vi "svx_Property Page.vi"(6 "Z Scale Graph Refnum":refnum<vi>, 7 "XY Graph Reference":refnum<vi>, 8 "XY Scale Graph Refnum":refnum<vi>, 9 "Container Refnum":refnum<vi>, 10 "State in":T1={"X Scale Width %"=50.0, "Y Scale Height %"=50.0, "X-Axis Range"={"Minimum"=0.0, "Maximum"=10.0}, "Y-Axis Range"={"Minimum"=0.0, "Maximum"=10.0}, "Z-Axis Range"={"Minimum"=0.0, "Maximum"=10.0}, "Plot Color"=61212, "Frame Color"=16252785, "Background Color"=16777222, "Initial AutoScale Y"=TRUE, "AutoScale X"=2, "AutoScale Y"=2, "AutoScale Z"=2, "Plot Transparency"=FALSE, "X-Axis Name"="Frequency", "Y-Axis Name"="Amplitude", "Z-Axis Name"="", "X-Axis Scaling Factor"={"Offset"=0.0, "Multiplier"=1.0}, "Y-Axis Scaling Factor"={"Offset"=0.0, "Multiplier"=1.0}, "Z-Axis Scaling Factor"={"Offset"=0.0, "Multiplier"=1.0}, "X-Scale Visible"=TRUE, "Y-Scale Visible"=TRUE, "Z-Scale Visible"=TRUE, "X-Scale Label Visible"=TRUE, "Y-Scale Label Visible"=TRUE, "Z-Scale Label Visible"=TRUE, "X-Axis Range Scaled"={"Minimum"=0.0, "Maximum"=10.0}, "Y-Axis Range Scaled"={"Minimum"=0.0, "Maximum"=10.0}, "Z-Axis Range Scaled"={"Minimum"=0.0, "Maximum"=10.0}, "Rev Z Order"=FALSE, "X-Scale Format Str"="%#.4g", "Y-Scale Format Str"="%#.4g", "Z-Scale Format Str"="%#.4g", "Decor color"=12369084, "Scale Range Change"=refnum, "out of state queue"=refnum, "property nodes"=refnum, "Lines"=[], "Line Properties"={"Line Color"=61212, "Line Width"=61212, "Line Style"=enum."Dash", "DisplayLines"=FALSE}} caption="State" {"Line Properties"."Line Width" min=1}, 11 "Data In":T3={"z0"=0.0, "dz"=1.0, "Plots"=[]}) -> (1 "Cancel?":bool, 2 "State out":T1={"X Scale Width %"=50.0, "Y Scale Height %"=50.0, "X-Axis Range"={"Minimum"=0.0, "Maximum"=10.0}, "Y-Axis Range"={"Minimum"=0.0, "Maximum"=10.0}, "Z-Axis Range"={"Minimum"=0.0, "Maximum"=10.0}, "Plot Color"=61212, "Frame Color"=16252785, "Background Color"=16777222, "Initial AutoScale Y"=TRUE, "AutoScale X"=2, "AutoScale Y"=2, "AutoScale Z"=2, "Plot Transparency"=FALSE, "X-Axis Name"="Frequency", "Y-Axis Name"="Amplitude", "Z-Axis Name"="", "X-Axis Scaling Factor"={"Offset"=0.0, "Multiplier"=1.0}, "Y-Axis Scaling Factor"={"Offset"=0.0, "Multiplier"=1.0}, "Z-Axis Scaling Factor"={"Offset"=0.0, "Multiplier"=1.0}, "X-Scale Visible"=TRUE, "Y-Scale Visible"=TRUE, "Z-Scale Visible"=TRUE, "X-Scale Label Visible"=TRUE, "Y-Scale Label Visible"=TRUE, "Z-Scale Label Visible"=TRUE, "X-Axis Range Scaled"={"Minimum"=0.0, "Maximum"=10.0}, "Y-Axis Range Scaled"={"Minimum"=0.0, "Maximum"=10.0}, "Z-Axis Range Scaled"={"Minimum"=0.0, "Maximum"=10.0}, "Rev Z Order"=FALSE, "X-Scale Format Str"="%#.4g", "Y-Scale Format Str"="%#.4g", "Z-Scale Format Str"="%#.4g", "Decor color"=12369084, "Scale Range Change"=refnum, "out of state queue"=refnum, "property nodes"=refnum, "Lines"=[], "Line Properties"={"Line Color"=61212, "Line Width"=61212, "Line Style"=enum."Dash", "DisplayLines"=FALSE}} caption="State" {"Line Properties"."Line Width" min=1})   [LabVIEW 2017, in "SVX Waterfall Graph.xctl"]
uses:
  <vilib>/addons/_XControls/Waterfall Graph/SVX Waterfall Graph.xctl
  <vilib>/addons/_XControls/Waterfall Graph/subVIs/svx_Waterfall Data.ctl
  <vilib>/addons/_XControls/Waterfall Graph/subVIs/svx_Waterfall State.ctl
  <vilib>/addons/_NISVFA/_Shared subVIs/Controls/svc_Cluster of Array of Cluster of XYZ.ctl
  <vilib>/addons/_XControls/Waterfall Graph/subVIs/svx_Waterfall Property Page User Events.ctl
panel:
  in  "Help":bool
  in  "Cancel":bool
  in  "OK":bool
  in  "Tab Control":T4(tab)
  in  "Reverse Order":bool
  in  "Plot Transparency":bool
  in  "Background color":u32(colorbox)
  in  "Frame color":u32(colorbox)
  in  "Plot color":u32(colorbox)
  in  "Enable State":T5(radio)
  in  "Caption":string
  in  "Label":string
  in  "Caption Visible?":bool
  in  "Label Visible?":bool
  in  "trailing zeros":bool
  in  "Digits":u8=1
  in  "Precision Type":u16(ring) caption="Precision type" items=["Digits of precision", "Significant digits"]
  in  "Type":i32(listbox)
  in  "FP Axis":enum16{"X-Axis", "Y-Axis", "Z-Axis"}(ring)
  in  "Scaling Factors - Multiplier":dbl caption="Multiplier"
  in  "Scaling Factors - Offset":dbl caption="Offset"
  in  "Range Maximum":dbl caption="Maximum"
  in  "Range Minimum":dbl caption="Minimum"
  in  "Autoscale":bool
  in  "Show Scale":bool
  in  "Show Scale label":bool
  in  "Scale Name":string caption="Name"
  in  "Scale Axis":enum16{"X-Axis", "Y-Axis", "Z-Axis"}(ring)
  in  "Line color":u32(colorbox)
  in  "Line width":u16=1 min=1 max=5
  in  "Style":T6(ring)=enum."Dash"
  in  "DisplayLines":bool
  in  "Tip strip":string
  in  "Description":string
  # "Label"
  # "Caption"
  # "Enabled State"
  # "Color Scheme"
  # "Scaling factors"
  # "Line Settings"
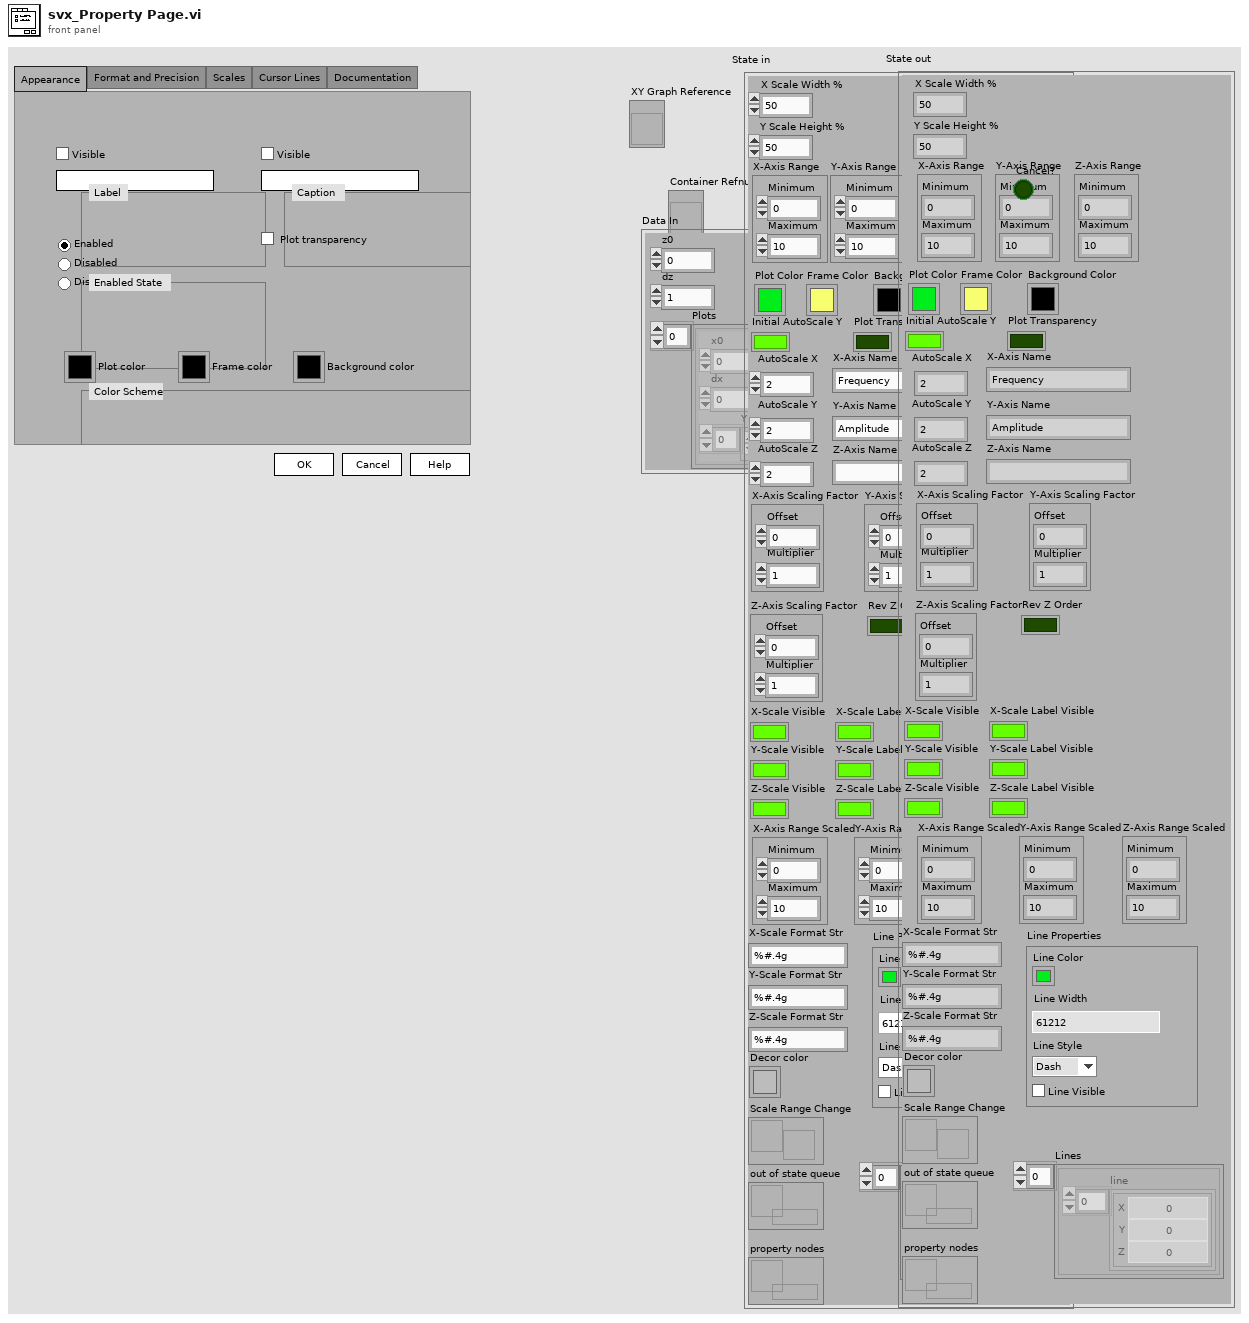
[diagram p1: front panel]
types:
  T1 = typedef "SVX Waterfall Graph.xctl/svx_Waterfall State.ctl" = cluster{"X Scale Width %":dbl, "Y Scale Height %":dbl, "X-Axis Range":cluster{"Minimum":dbl, "Maximum":dbl}, "Y-Axis Range":cluster{"Minimum":dbl, "Maximum":dbl}, "Z-Axis Range":cluster{"Minimum":dbl, "Maximum":dbl}, "Plot Color":u32, "Frame Color":u32, "Background Color":u32, "Initial AutoScale Y":bool, "AutoScale X":u8, "AutoScale Y":u8, "AutoScale Z":u8, "Plot Transparency":bool, "X-Axis Name":string, "Y-Axis Name":string, "Z-Axis Name":string, "X-Axis Scaling Factor":cluster{"Offset":dbl, "Multiplier":dbl}, "Y-Axis Scaling Factor":cluster{"Offset":dbl, "Multiplier":dbl}, "Z-Axis Scaling Factor":cluster{"Offset":dbl, "Multiplier":dbl}, "X-Scale Visible":bool, "Y-Scale Visible":bool, "Z-Scale Visible":bool, "X-Scale Label Visible":bool, "Y-Scale Label Visible":bool, "Z-Scale Label Visible":bool, "X-Axis Range Scaled":cluster{"Minimum":dbl, "Maximum":dbl}, "Y-Axis Range Scaled":cluster{"Minimum":dbl, "Maximum":dbl}, "Z-Axis Range Scaled":cluster{"Minimum":dbl, "Maximum":dbl}, "Rev Z Order":bool, "X-Scale Format Str":string, "Y-Scale Format Str":string, "Z-Scale Format Str":string, "Decor color":u32, "Scale Range Change":refnum<user-event>, "out of state queue":refnum<queue>, "property nodes":refnum<queue>, "Lines":T2[], "Line Properties":cluster{"Line Color":u32, "Line Width":u16, "Line Style":enum32{"Solid", "Dash", "Dot", "DashDot", "DashDotDot"}, "DisplayLines":bool}}
  T2 = typedef "svc_Cluster of Array of Cluster of XYZ.ctl" = cluster{"line":cluster{"X":dbl, "Y":dbl, "Z":dbl}[]}
  T3 = typedef "SVX Waterfall Graph.xctl/svx_Waterfall Data.ctl" = cluster{"z0":dbl, "dz":dbl, "Plots":cluster{"x0":dbl, "dx":dbl, "Y":dbl[]}[]}
  T4 = enum32{"Appearance", "Format and Precision", "Scales", "Cursor Lines", "Documentation"}
  T5 = enum32{"Enabled", "Disabled", "Disabled & grayed"}
  T6 = enum32{"Solid", "Dash", "Dot", "DashDot", "DashDotDot"}
  T7 = typedef "SVX Waterfall Graph.xctl/svx_Waterfall Property Page User Events.ctl" = enum16{"Redraw Frame", "Update Graph", "Exit"}
  T8 = cluster{"Container Changed":bool, "Scales Changed":bool, "Waveform Changed":bool}
  T9 = cluster{"Line Color":u32, "Line Width":u16, "Line Style":enum32{"Solid", "Dash", "Dot", "DashDot", "DashDotDot"}, "DisplayLines":bool}
  T10 = cluster{"Label.Text":string, "Label.Visible":bool, "Caption.Text":string, "Caption.Visible":bool, "Disabled":u8, "Desc":string, "TipStrip":string}
  T11 = cluster{"Width":u16, "Style":enum32{"Solid", "Dash", "Dot", "DashDot", "DashDotDot"}}
  T12 = typedef "SVX Waterfall Graph.xctl/svx_CroppedData.ctl" = cluster{"Dec/Cropped in":T3, "Lines":T2[]}
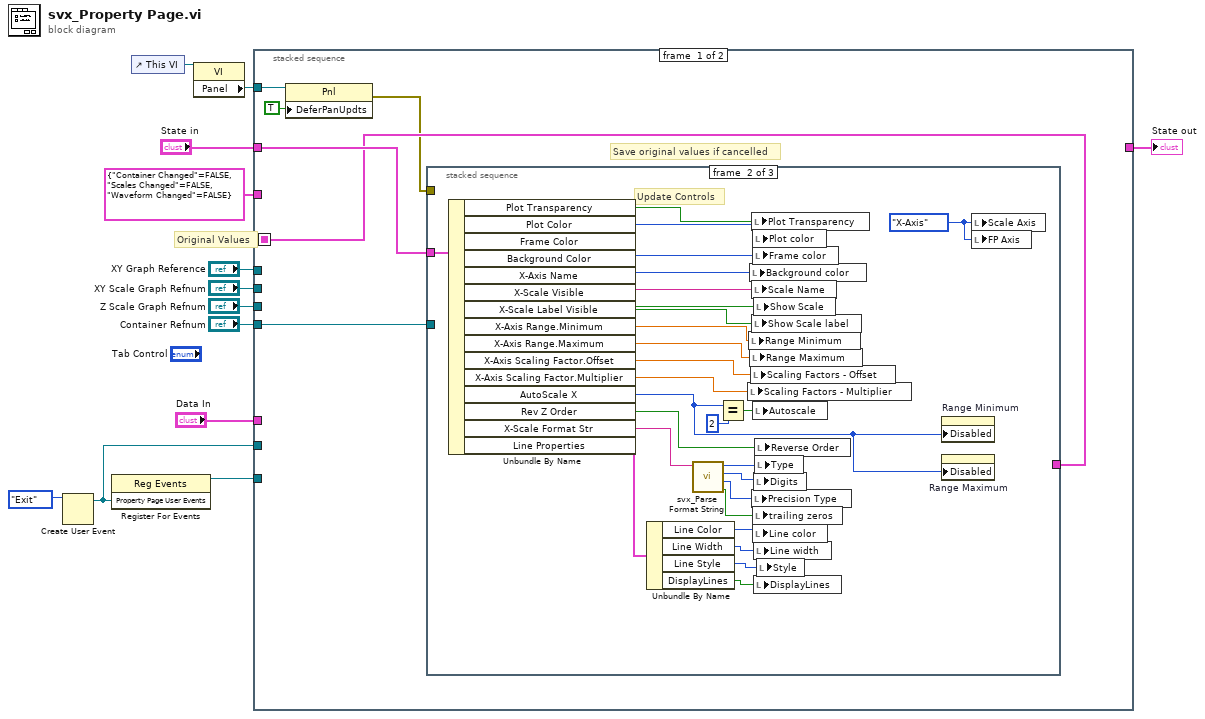
[diagram p0: block diagram]
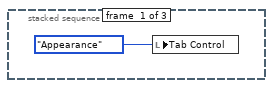
[diagram p2: hidden frame]
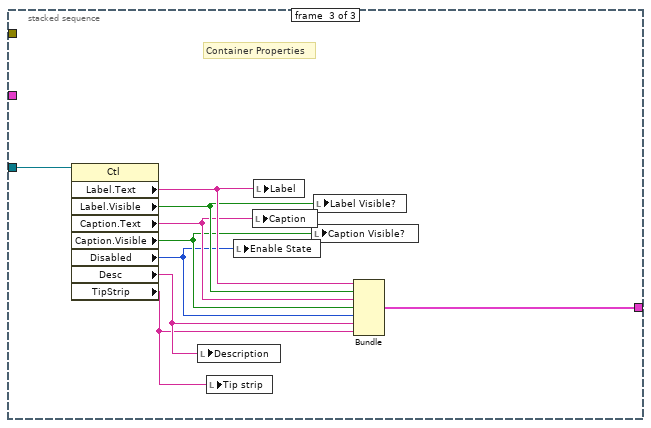
[diagram p3: hidden frame]
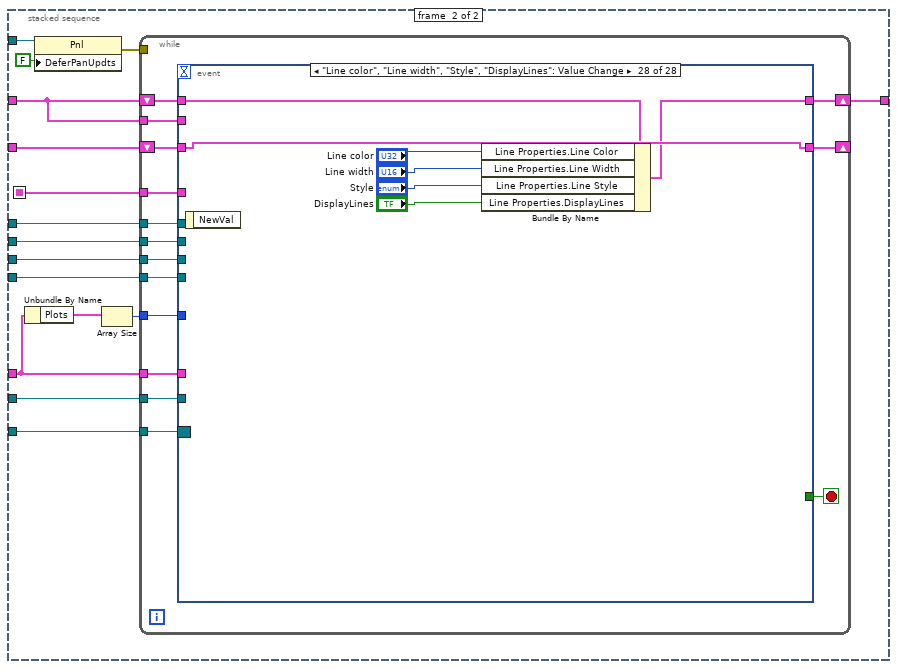
[diagram p4: hidden frame]
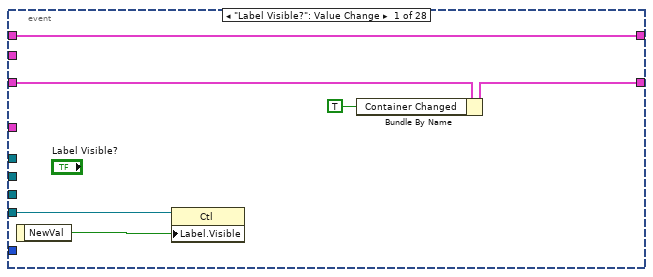
[diagram p5: hidden frame]
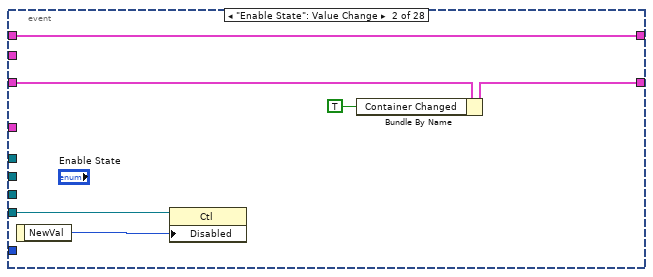
[diagram p6: hidden frame]
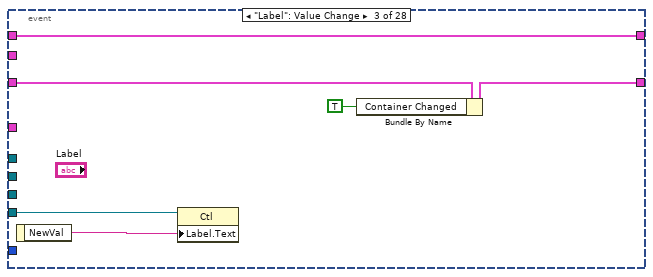
[diagram p7: hidden frame]
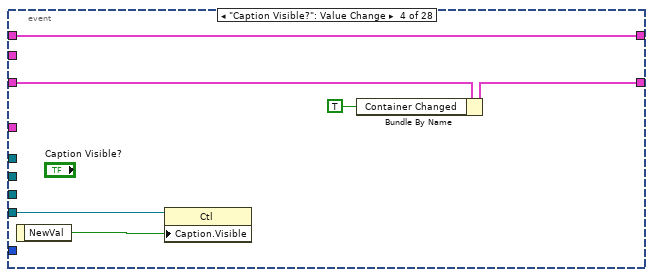
[diagram p8: hidden frame]
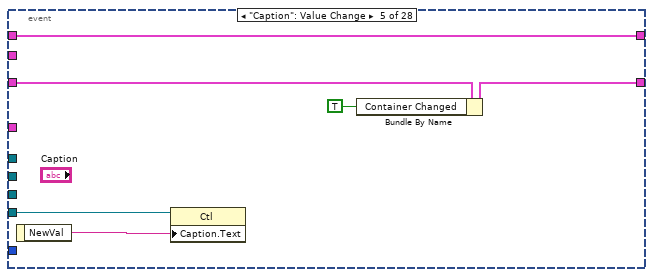
[diagram p9: hidden frame]
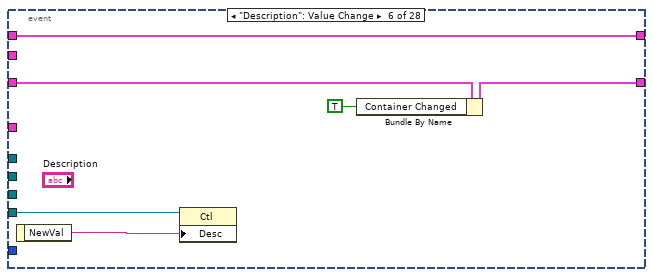
[diagram p10: hidden frame]
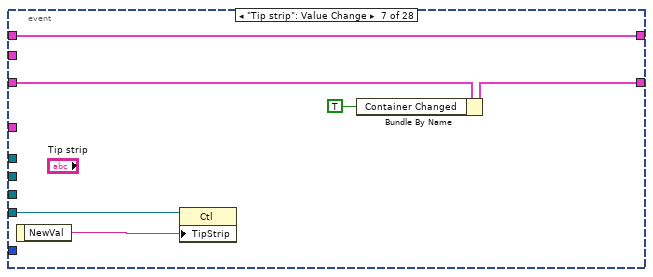
[diagram p11: hidden frame]
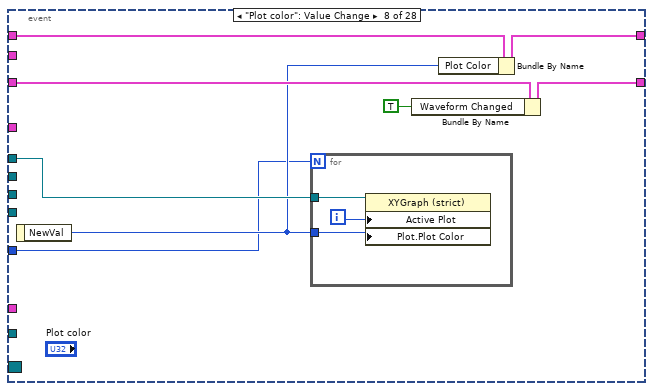
[diagram p12: hidden frame]
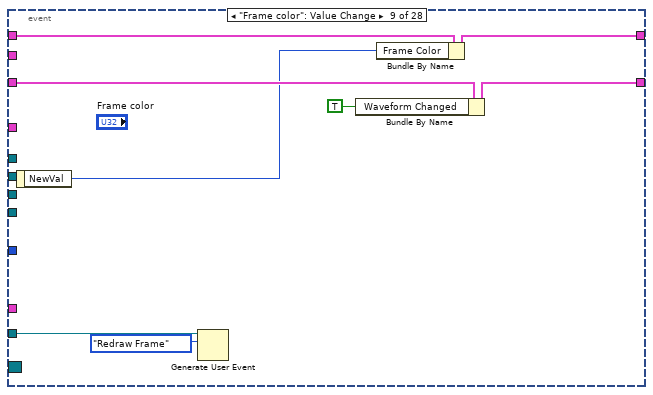
[diagram p13: hidden frame]
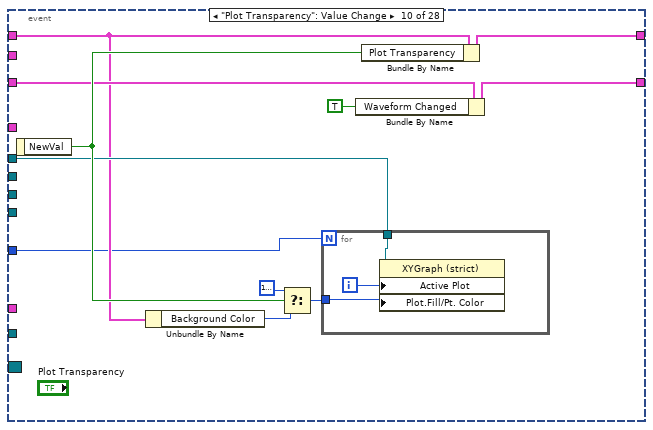
[diagram p14: hidden frame]
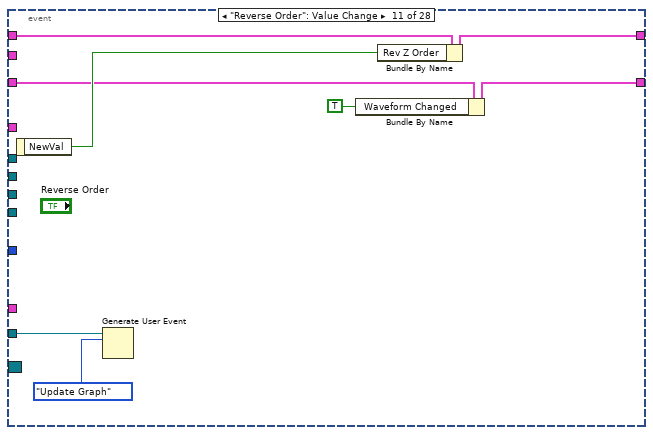
[diagram p15: hidden frame]
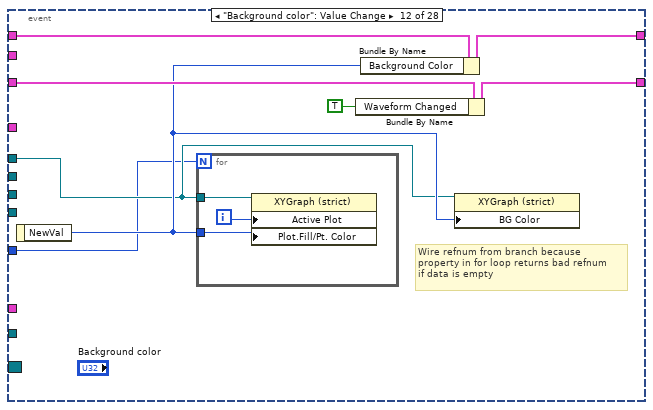
[diagram p16: hidden frame]
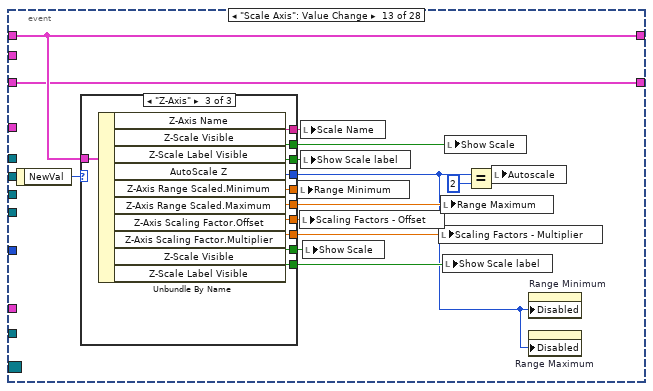
[diagram p17: hidden frame]
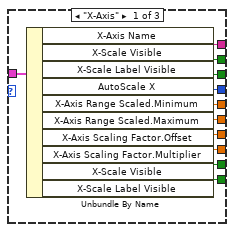
[diagram p18: hidden frame]
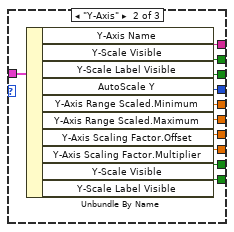
[diagram p19: hidden frame]
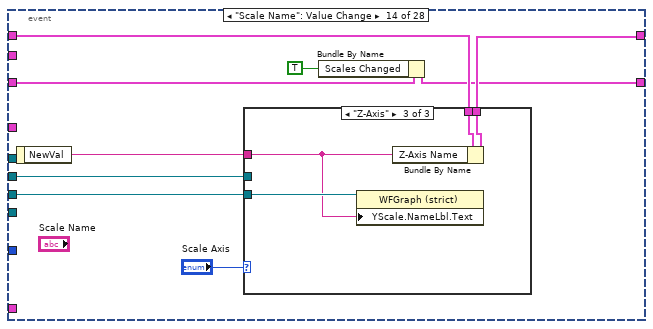
[diagram p20: hidden frame]
diagram:
  # "Original Values"
  n1 = Create User Event(user event datatype=svx_Waterfall_Property_Page_User_Events."Exit" ("Property Page User Events")) -> (user event=w4:refnum<user-event>)  [unwired: 1 in, 1 out]
  n2 = register-events(w4) -> (reference out=w6:refnum<event-registration>)  [unwired: 2 in, 1 out]
  n3 = control-ref of="This VI"() -> (w2:refnum<vi>)
  n4 = property class="VI"(reference=w2) -> ("Panel"=w1:refnum<vi>)  [unwired: 1 in, 2 out]
  n5 = stacked-sequence {
    seq-local: [w17 _] -> [_ w65]
    tunnel: T8 {"Container Changed"=FALSE, "Scales Changed"=FALSE, "Waveform Changed"=FALSE} -> [_ w72]
    tunnel: "XY Graph Reference" -> [_ w71]
    tunnel: "XY Scale Graph Refnum" -> [_ w70]
    tunnel: "Z Scale Graph Refnum" -> [_ w69]
    tunnel: "Container Refnum" -> [w19 w68]
    tunnel: "State in" -> [w18 w66]
    tunnel: [_ w67] -> w8
    tunnel: "Data In" -> [_ w58]
    tunnel: w6 -> [_ w64]
    tunnel: w4 -> [_ w63]
    tunnel: w1 -> [w16 w61]
    frame #0 {
      # "Save original values if cancelled"
      n6 = property class="Pnl"(reference=w16, "DeferPanUpdts"=TRUE ("Defer Panel Updates")) -> (error out=w14:errorcluster)  [unwired: 1 in, 1 out]
      n7 = stacked-sequence {
        tunnel: w19 -> [_ _ w56]
        tunnel: [_ _ w55] -> w17
        tunnel: w18 -> [_ w47 _]
        tunnel: w14 -> [_ _ _]
        frame #0 {
          n8 = local write "Tab Control"(T4."Appearance" ("Tab Control")) -> ()
        }
        frame #1 {
          w32 = enum16{"X-Axis", "Y-Axis", "Z-Axis"}."X-Axis" ("Axis")
          # "Update Controls"
          n9 = Unbundle By Name(w47) -> ("Plot Transparency"=w37:bool, "Plot Color"=w46:u32, "Frame Color"=w45:u32, "Background Color"=w44:u32, "X-Axis Name"=w43:string, "X-Scale Visible"=w42:bool, "X-Scale Label Visible"=w41:bool, "X-Axis Range.Minimum"=w40:dbl, "X-Axis Range.Maximum"=w26:dbl, "X-Axis Scaling Factor.Offset"=w39:dbl, "X-Axis Scaling Factor.Multiplier"=w38:dbl, "AutoScale X"=w36:u8, "Rev Z Order"=w33:bool, "X-Scale Format Str"=w31:string, "Line Properties"=w25:T9)
          n10 = Unbundle By Name(w25) -> ("Line Color"=w24:u32, "Line Width"=w23:u16, "Line Style"=w22:T6, "DisplayLines"=w21:bool)
          n11 = call <vilib>:"svx_Parse Format String.vi"("Format string"=w31) -> ("trailing zeros"=w27:bool, "Precision Type"=w28:u16, "Digits"=w29:u8, "Type"=w30:i32)  [unwired: 6 in, 1 out]
          n12 = Equal?(x=w36, y=u8 2) -> (x = y?=w34:bool)
          n13 = local write "Scaling Factors - Multiplier"(w38) -> ()
          n14 = local write "Range Minimum"(w40) -> ()
          n15 = local write "Background color"(w44) -> ()
          n16 = local write "Range Maximum"(w26) -> ()
          n17 = local write "Scaling Factors - Offset"(w39) -> ()
          n18 = local write "Plot Transparency"(w37) -> ()
          n19 = local write "Scale Name"(w43) -> ()
          n20 = local write "Show Scale label"(w41) -> ()
          n21 = local write "Precision Type"(w28) -> ()
          n22 = local write "Plot color"(w46) -> ()
          n23 = local write "Frame color"(w45) -> ()
          n24 = local write "Autoscale"(w34) -> ()
          n25 = local write "trailing zeros"(w27) -> ()
          n26 = local write "Line color"(w24) -> ()
          n27 = local write "Show Scale"(w42) -> ()
          n28 = local write "Digits"(w29) -> ()
          n29 = local write "Line width"(w23) -> ()
          n30 = local write "DisplayLines"(w21) -> ()
          n31 = local write "Reverse Order"(w33) -> ()
          n32 = local write "Type"(w30) -> ()
          n33 = local write "Style"(w22) -> ()
          n34 = property on="Range Minimum" class="DigNum (strict)"("Disabled"=w36) -> ()  [unwired: 2 in, 2 out]
          n35 = property on="Range Maximum" class="DigNum (strict)"("Disabled"=w36) -> ()  [unwired: 2 in, 2 out]
          n36 = local write "Scale Axis"(w32) -> ()
          n37 = local write "FP Axis"(w32) -> ()
        }
        frame #2 {
          # "Container Properties"
          n38 = property class="Ctl"(reference=w56) -> ("Label.Text"=w54:string, "Label.Visible"=w53:bool, "Caption.Text"=w52:string, "Caption.Visible"=w51:bool, "Disabled"=w50:u8, "Desc"=w49:string, "TipStrip"=w48:string)  [unwired: 1 in, 2 out]
          n39 = local write "Description"(w49) -> ()
          n40 = local write "Tip strip"(w48) -> ()
          n41 = local write "Enable State"(w50) -> ()
          n42 = local write "Caption"(w52) -> ()
          n43 = local write "Label"(w54) -> ()
          n44 = local write "Caption Visible?"(w51) -> ()
          n45 = local write "Label Visible?"(w53) -> ()
          n46 = Bundle("Label.Text"=w54, "Label.Visible"=w53, "Caption.Text"=w52, "Caption.Visible"=w51, "Disabled"=w50, "Desc"=w49, "TipStrip"=w48) -> (w55:T10)  [unwired: 1 in]
        }
      }
    }
    frame #1 {
      n47 = Unbundle By Name(w58) -> ("Plots"=w59:cluster{"x0":dbl, "dx":dbl, "Y":dbl[]}[])
      n48 = property class="Pnl"(reference=w61, "DeferPanUpdts"=FALSE ("Defer Panel Updates")) -> (error out=w60:errorcluster)  [unwired: 1 in, 1 out]
      n49 = Array Size(array=w59) -> (size(s)=w57:i32)
      n50 = while {
        shift-right: [w85] -> _
        shift-left: w72 -> [w86]
        tunnel: w71 -> [w84]
        tunnel: w70 -> [w83]
        tunnel: w69 -> [w82]
        tunnel: w68 -> [w81]
        shift-right: [w79] -> w67
        shift-left: w66 -> [w80]
        tunnel: w66 -> [w78]
        tunnel: w65 -> [w77]
        tunnel: w58 -> [w76]
        tunnel: w64 -> [w75]
        tunnel: w63 -> [w74]
        tunnel: w60 -> [_]
        tunnel: w57 -> [w73]
        stop <- w87 stop-if-true
        n51 = event shown="[27] \"Line color\", \"Line width\", \"Style\", \"DisplayLines\": Value Change" {
          selector: w75 -> [_ _ _ _ _ _ _ _ _ _ _ _ _ _ _ _ _ _ _ _ _ _ _ _ _ _ _ _]
          dyn-events: _ -> [_ _ _ _ _ _ _ _ _ _ _ _ _ _ _ _ _ _ _ _ _ _ _ _ _ _ _ _]
          timeout: _ -> [_ _ _ _ _ _ _ _ _ _ _ _ _ _ _ _ _ _ _ _ _ _ _ _ _ _ _ _]
          tunnel: [_ _ _ _ _ _ _ _ _ _ _ _ _ _ _ _ _ _ _ _ _ _ _ w556 _ _ w652 _] -> w87
          tunnel: w86 -> [w93 w99 w105 w111 w117 w123 w129 w137 w148 w153 w166 w178 w187 w231 w253 w274 w295 w346 w403 w451 w502 w521 w542 w560 w569 w644 w654 w734]
          tunnel: [w92 w98 w104 w110 w116 w122 w128 w136 w147 w159 w170 w177 w187 w230 w252 w273 w294 w345 w402 w450 w501 w521 w541 w560 w569 w644 w654 w734] -> w85
          tunnel: w84 -> [_ _ _ _ _ _ _ w134 _ w151 _ w172 _ _ _ _ _ _ w407 w455 _ _ _ _ w565 _ w651 _]
          tunnel: w83 -> [_ _ _ _ _ _ _ _ _ _ _ _ _ w234 w256 w277 w301 w352 w410 w458 _ _ w537 _ w563 _ w650 _]
          tunnel: w82 -> [_ _ _ _ _ _ _ _ _ _ _ _ _ w233 w255 w276 w300 w351 w409 w457 _ _ w536 _ w562 _ w646 _]
          tunnel: w81 -> [w90 w96 w102 w108 w114 w120 w126 _ _ _ _ _ _ _ _ _ _ _ _ _ _ _ _ _ w568 _ _ _]
          tunnel: w80 -> [w88 w94 w100 w106 w112 w118 w124 w133 w145 w150 w165 w175 w195 w238 w259 w280 w304 w355 w413 w461 w507 w518 w539 w559 _ w643 w648 w733]
          tunnel: [w88 w94 w100 w106 w112 w118 w124 w132 w144 w157 w168 w174 w195 w237 w258 w279 w303 w354 w412 w460 w506 w518 w540 w559 w566 w643 w645 w732] -> w79
          tunnel: w78 -> [_ _ _ _ _ _ _ _ _ _ _ _ _ _ _ _ _ _ _ _ _ _ _ _ w566 _ _ _]
          tunnel: w77 -> [_ _ _ _ _ _ _ _ _ _ _ _ _ _ _ _ _ _ _ _ _ _ _ _ w564 _ _ _]
          tunnel: w76 -> [_ _ _ _ _ _ _ _ _ _ _ _ _ _ _ _ _ _ _ _ _ _ _ _ _ _ w649 _]
          tunnel: w74 -> [_ _ _ _ _ _ _ _ w142 _ w163 _ _ _ _ _ w293 w344 w406 w454 w505 _ _ w557 w567 _ w647 _]
          tunnel: w73 -> [_ _ _ _ _ _ _ w130 _ w149 _ w171 _ _ _ _ _ _ _ _ _ _ _ _ w561 _ _ _]
          event "Label Visible?": Value Change {
            n52 = event-data() -> ("NewVal"=w89:bool)  [unwired: 1 in]
            n53 = property class="Ctl"(reference=w90, "Label.Visible"=w89) -> ()  [unwired: 1 in, 2 out]
            n54 = Bundle By Name(cluster=w93, "Container Changed"=TRUE) -> (w92:T8)
          }
          event "Enable State": Value Change {
            n55 = event-data() -> ("NewVal"=w95:T5)  [unwired: 1 in]
            n56 = property class="Ctl"(reference=w96, "Disabled"=w95) -> ()  [unwired: 1 in, 2 out]
            n57 = Bundle By Name(cluster=w99, "Container Changed"=TRUE) -> (w98:T8)
          }
          event "Label": Value Change {
            n58 = event-data() -> ("NewVal"=w101:string)  [unwired: 1 in]
            n59 = property class="Ctl"(reference=w102, "Label.Text"=w101) -> ()  [unwired: 1 in, 2 out]
            n60 = Bundle By Name(cluster=w105, "Container Changed"=TRUE) -> (w104:T8)
          }
          event "Caption Visible?": Value Change {
            n61 = event-data() -> ("NewVal"=w107:bool)  [unwired: 1 in]
            n62 = property class="Ctl"(reference=w108, "Caption.Visible"=w107) -> ()  [unwired: 1 in, 2 out]
            n63 = Bundle By Name(cluster=w111, "Container Changed"=TRUE) -> (w110:T8)
          }
          event "Caption": Value Change {
            n64 = event-data() -> ("NewVal"=w113:string)  [unwired: 1 in]
            n65 = property class="Ctl"(reference=w114, "Caption.Text"=w113) -> ()  [unwired: 1 in, 2 out]
            n66 = Bundle By Name(cluster=w117, "Container Changed"=TRUE) -> (w116:T8)
          }
          event "Description": Value Change {
            n67 = event-data() -> ("NewVal"=w119:string)  [unwired: 1 in]
            n68 = property class="Ctl"(reference=w120, "Desc"=w119) -> ()  [unwired: 1 in, 2 out]
            n69 = Bundle By Name(cluster=w123, "Container Changed"=TRUE) -> (w122:T8)
          }
          event "Tip strip": Value Change {
            n70 = event-data() -> ("NewVal"=w125:string)  [unwired: 1 in]
            n71 = property class="Ctl"(reference=w126, "TipStrip"=w125) -> ()  [unwired: 1 in, 2 out]
            n72 = Bundle By Name(cluster=w129, "Container Changed"=TRUE) -> (w128:T8)
          }
          event "Plot color": Value Change {
            n73 = event-data() -> ("NewVal"=w131:u32)  [unwired: 1 in]
            n74 = for {
              N: w130 -> [_]
              tunnel: w131 -> [w139]
              tunnel: w134 -> [w140]
              i -> [w138]
              n75 = property class="XYGraph (strict)"(reference=w140, "Active Plot"=w138, "Plot.Plot Color"=w139) -> ()  [unwired: 1 in, 2 out]
            }
            n76 = Bundle By Name(cluster=w137, "Waveform Changed"=TRUE ("Container Changed")) -> (w136:T8)
            n77 = Bundle By Name(cluster=w133, "Plot Color"=w131) -> (w132:T1)
          }
          event "Frame color": Value Change {
            n78 = event-data() -> ("NewVal"=w143:u32)  [unwired: 1 in]
            n79 = Generate User Event(user event=w142, event data cluster=svx_Waterfall_Property_Page_User_Events."Redraw Frame" ("Property Page User Events")) -> ()  [unwired: 2 in, 2 out]
            n80 = Bundle By Name(cluster=w148, "Waveform Changed"=TRUE ("Container Changed")) -> (w147:T8)
            n81 = Bundle By Name(cluster=w145, "Frame Color"=w143) -> (w144:T1)
          }
          event "Plot Transparency": Value Change {
            n82 = event-data() -> ("NewVal"=w155:bool)  [unwired: 1 in]
            n83 = Unbundle By Name(w150) -> ("Background Color"=w152:u32)
            n84 = Select(t=u32 16777216, s=w155, f=w152) -> (s? t:f=w156:u32)
            n85 = for {
              N: w149 -> [_]
              tunnel: w156 -> [w161]
              tunnel: w151 -> [w160]
              i -> [w162]
              n86 = property on="Property Node" class="XYGraph (strict)"(reference=w160, "Active Plot"=w162, "Plot.Fill/Pt. Color"=w161) -> ()  [unwired: 1 in, 2 out]
            }
            n87 = Bundle By Name(cluster=w153, "Waveform Changed"=TRUE) -> (w159:T8)
            n88 = Bundle By Name(cluster=w150, "Plot Transparency"=w155) -> (w157:T1)
          }
          event "Reverse Order": Value Change {
            n89 = event-data() -> ("NewVal"=w167:bool)  [unwired: 1 in]
            n90 = Generate User Event(user event=w163, event data cluster=svx_Waterfall_Property_Page_User_Events."Update Graph" ("event data")) -> ()  [unwired: 2 in, 2 out]
            n91 = Bundle By Name(cluster=w166, "Waveform Changed"=TRUE) -> (w170:T8)
            n92 = Bundle By Name(cluster=w165, "Rev Z Order"=w167) -> (w168:T1)
          }
          event "Background color": Value Change {
            # "Wire refnum from branch because\nproperty in for loop returns bad refnum\nif data is empty"
            n93 = event-data() -> ("NewVal"=w173:u32)  [unwired: 1 in]
            n94 = for {
              N: w171 -> [_]
              tunnel: w173 -> [w180]
              tunnel: w172 -> [w181]
              i -> [w179]
              n95 = property class="XYGraph (strict)"(reference=w181, "Active Plot"=w179, "Plot.Fill/Pt. Color"=w180) -> ()  [unwired: 1 in, 2 out]
            }
            n96 = Bundle By Name(cluster=w178, "Waveform Changed"=TRUE ("Container Changed")) -> (w177:T8)
            n97 = Bundle By Name(cluster=w175, "Background Color"=w173) -> (w174:T1)
            n98 = property class="XYGraph (strict)"(reference=w172, "BG Color"=w173) -> ()  [unwired: 1 in, 2 out]
          }
          event "Scale Axis": Value Change {
            n99 = event-data() -> ("NewVal"=w196:enum16{"X-Axis", "Y-Axis", "Z-Axis"})  [unwired: 1 in]
            n100 = case shown="\"Z-Axis\"" w196 {
              tunnel: w195 -> [w207 w218 w229]
              tunnel: [w206 w217 w228] -> w184
              tunnel: [w205 w216 w227] -> w194
              tunnel: [w204 w215 w226] -> w193
              tunnel: [w203 w214 w225] -> w192
              tunnel: [w202 w213 w224] -> w191
              tunnel: [w201 w212 w223] -> w190
              tunnel: [w200 w211 w222] -> w189
              tunnel: [w199 w210 w221] -> w188
              tunnel: [w198 w209 w220] -> w186
              tunnel: [w197 w208 w219] -> w185
              frame "X-Axis" {
                n101 = Unbundle By Name(w207) -> ("X-Axis Name"=w199:string, "X-Scale Visible"=w200:bool, "X-Scale Label Visible"=w201:bool, "AutoScale X"=w206:u8, "X-Axis Range Scaled.Minimum"=w205:dbl, "X-Axis Range Scaled.Maximum"=w204:dbl, "X-Axis Scaling Factor.Offset"=w203:dbl, "X-Axis Scaling Factor.Multiplier"=w202:dbl, "X-Scale Visible"=w198:bool, "X-Scale Label Visible"=w197:bool)
              }
              frame "Y-Axis" {
                n102 = Unbundle By Name(w218) -> ("Y-Axis Name"=w210:string, "Y-Scale Visible"=w211:bool, "Y-Scale Label Visible"=w212:bool, "AutoScale Y"=w217:u8, "Y-Axis Range Scaled.Minimum"=w216:dbl, "Y-Axis Range Scaled.Maximum"=w215:dbl, "Y-Axis Scaling Factor.Offset"=w214:dbl, "Y-Axis Scaling Factor.Multiplier"=w213:dbl, "Y-Scale Visible"=w209:bool, "Y-Scale Label Visible"=w208:bool)
              }
              frame "Z-Axis" {
                n103 = Unbundle By Name(w229) -> ("Z-Axis Name"=w221:string, "Z-Scale Visible"=w222:bool, "Z-Scale Label Visible"=w223:bool, "AutoScale Z"=w228:u8, "Z-Axis Range Scaled.Minimum"=w227:dbl, "Z-Axis Range Scaled.Maximum"=w226:dbl, "Z-Axis Scaling Factor.Offset"=w225:dbl, "Z-Axis Scaling Factor.Multiplier"=w224:dbl, "Z-Scale Visible"=w220:bool, "Z-Scale Label Visible"=w219:bool)
              }
            }
            n104 = local write "Range Minimum"(w194) -> ()
            n105 = local write "Scaling Factors - Offset"(w192) -> ()
            n106 = local write "Scale Name"(w188) -> ()
            n107 = local write "Show Scale label"(w190) -> ()
            n108 = local write "Show Scale"(w186) -> ()
            n109 = local write "Scaling Factors - Multiplier"(w191) -> ()
            n110 = local write "Range Maximum"(w193) -> ()
            n111 = local write "Show Scale label"(w185) -> ()
            n112 = local write "Show Scale"(w189) -> ()
            n113 = Equal?(x=w184, y=u8 2) -> (x = y?=w182:bool)
            n114 = local write "Autoscale"(w182) -> ()
            n115 = property on="Range Minimum" class="DigNum (strict)"("Disabled"=w184) -> ()  [unwired: 2 in, 2 out]
            n116 = property on="Range Maximum" class="DigNum (strict)"("Disabled"=w184) -> ()  [unwired: 2 in, 2 out]
          }
          event "Scale Name": Value Change {
            n117 = event-data() -> ("NewVal"=w235:string)  [unwired: 1 in]
            n118 = case shown="\"Z-Axis\"" "Scale Axis" {
              tunnel: w238 -> [w242 w246 w250]
              tunnel: [w241 w245 w249] -> w237
              tunnel: w235 -> [w240 w243 w247]
              tunnel: w234 -> [w239 w244 _]
              tunnel: w233 -> [_ _ w248]
              frame "X-Axis" {
                n119 = property class="WFGraph (strict)"(reference=w239, "XScale.NameLbl.Text"=w240) -> ()  [unwired: 1 in, 2 out]
                n120 = Bundle By Name(cluster=w242, "X-Axis Name"=w240) -> (w241:T1)
              }
              frame "Y-Axis" {
                n121 = property class="WFGraph (strict)"(reference=w244, "YScale.NameLbl.Text"=w243) -> ()  [unwired: 1 in, 2 out]
                n122 = Bundle By Name(cluster=w246, "Y-Axis Name"=w243) -> (w245:T1)
              }
              frame "Z-Axis" {
                n123 = property class="WFGraph (strict)"(reference=w248, "YScale.NameLbl.Text"=w247) -> ()  [unwired: 1 in, 2 out]
                n124 = Bundle By Name(cluster=w250, "Z-Axis Name"=w247) -> (w249:T1)
              }
            }
            n125 = Bundle By Name(cluster=w231, "Scales Changed"=TRUE) -> (w230:T8)
          }
          event "Show Scale": Value Change {
            n126 = event-data() -> ("NewVal"=w257:bool)  [unwired: 1 in]
            n127 = local read "Scale Axis"() -> (w251:enum16{"X-Axis", "Y-Axis", "Z-Axis"})
            n128 = case shown="\"Y-Axis\"" w251 {
              tunnel: w259 -> [w263 w267 w271]
              tunnel: [w262 w266 w270] -> w258
              tunnel: w257 -> [w261 w264 w268]
              tunnel: w256 -> [w260 w265 _]
              tunnel: w255 -> [_ _ w269]
              frame "X-Axis" {
                n129 = property class="WFGraph (strict)"(reference=w260, "XScale.Visible"=w261) -> ()  [unwired: 1 in, 2 out]
                n130 = Bundle By Name(cluster=w263, "X-Scale Visible"=w261) -> (w262:T1)
              }
              frame "Y-Axis" {
                n131 = property class="WFGraph (strict)"(reference=w265, "YScale.Visible"=w264) -> ()  [unwired: 1 in, 2 out]
                n132 = Bundle By Name(cluster=w267, "Y-Scale Visible"=w264) -> (w266:T1)
              }
              frame "Z-Axis" {
                n133 = property class="WFGraph (strict)"(reference=w269, "YScale.Visible"=w268) -> ()  [unwired: 1 in, 2 out]
                n134 = Bundle By Name(cluster=w271, "Z-Scale Visible"=w268) -> (w270:T1)
              }
            }
            n135 = Bundle By Name(cluster=w253, "Scales Changed"=TRUE) -> (w252:T8)
          }
          event "Show Scale label": Value Change {
            n136 = event-data() -> ("NewVal"=w278:bool)  [unwired: 1 in]
            n137 = local read "Scale Axis"() -> (w272:enum16{"X-Axis", "Y-Axis", "Z-Axis"})
            n138 = case shown="\"X-Axis\"" w272 {
              tunnel: w280 -> [w284 w288 w292]
              tunnel: [w283 w287 w291] -> w279
              tunnel: w278 -> [w282 w285 w289]
              tunnel: w277 -> [w281 w286 _]
              tunnel: w276 -> [_ _ w290]
              frame "X-Axis" {
                n139 = Bundle By Name(cluster=w284, "X-Scale Label Visible"=w282) -> (w283:T1)
                n140 = property class="WFGraph (strict)"(reference=w281, "XScale.NameLbl.Visible"=w282) -> ()  [unwired: 1 in, 2 out]
              }
              frame "Y-Axis" {
                n141 = Bundle By Name(cluster=w288, "Y-Scale Label Visible"=w285) -> (w287:T1)
                n142 = property class="WFGraph (strict)"(reference=w286, "YScale.NameLbl.Visible"=w285) -> ()  [unwired: 1 in, 2 out]
              }
              frame "Z-Axis" {
                n143 = Bundle By Name(cluster=w292, "Z-Scale Label Visible"=w289) -> (w291:T1)
                n144 = property class="WFGraph (strict)"(reference=w290, "YScale.NameLbl.Visible"=w289) -> ()  [unwired: 1 in, 2 out]
              }
            }
            n145 = Bundle By Name(cluster=w274, "Scales Changed"=TRUE) -> (w273:T8)
          }
          event "Scaling Factors - Offset": Value Change {
            n146 = local read "Scale Axis"() -> (w299:enum16{"X-Axis", "Y-Axis", "Z-Axis"})
            n147 = event-data() -> ("NewVal"=w302:dbl)  [unwired: 1 in]
            n148 = case shown="\"X-Axis\"" w299 {
              tunnel: w304 -> [w314 w327 w342]
              tunnel: [w315 w328 w343] -> w303
              tunnel: w302 -> [w308 w321 w336]
              tunnel: w301 -> [w305 w320 _]
              tunnel: w300 -> [_ _ w335]
              tunnel: [w307 w317 w331] -> w298
              tunnel: [w306 w316 w330] -> w297
              tunnel: w293 -> [_ _ w333]
              frame "X-Axis" {
                n149 = Unbundle By Name(w314) -> ("X-Axis Range.Minimum"=w313:dbl, "X-Axis Scaling Factor.Multiplier"=w310:dbl, "X-Axis Range.Maximum"=w311:dbl)
                n150 = Multiply(x=w313, y=w310) -> (x*y=w312:dbl)
                n151 = Multiply(x=w310, y=w311) -> (x*y=w309:dbl)
                n152 = Add(x=w308, y=w312) -> (x+y=w307:dbl)
                n153 = Add(x=w308, y=w309) -> (x+y=w306:dbl)
                n154 = Bundle By Name(cluster=w314, "X-Axis Scaling Factor.Offset"=w308, "X-Axis Range Scaled.Minimum"=w307, "X-Axis Range Scaled.Maximum"=w306) -> (w315:T1)
                n155 = property class="WFGraph (strict)"(reference=w305, "XScale.Minimum"=w307, "XScale.Maximum"=w306) -> ()  [unwired: 1 in, 2 out]
              }
              frame "Y-Axis" {
                n156 = Unbundle By Name(w327) -> ("Y-Axis Range.Minimum"=w326:dbl, "Y-Axis Scaling Factor.Multiplier"=w323:dbl, "Y-Axis Range.Maximum"=w324:dbl)
                n157 = Multiply(x=w326, y=w323) -> (x*y=w325:dbl)
                n158 = Multiply(x=w323, y=w324) -> (x*y=w322:dbl)
                n159 = Add(x=w321, y=w325) -> (x+y=w319:dbl)
                n160 = Add(x=w321, y=w322) -> (x+y=w318:dbl)
                n161 = Max & Min(x=w319, y=w318) -> (max(x,y)=w316:dbl, min(x,y)=w317:dbl)
                n162 = Bundle By Name(cluster=w327, "Y-Axis Scaling Factor.Offset"=w321, "Y-Axis Range Scaled.Minimum"=w317, "Y-Axis Range Scaled.Maximum"=w316) -> (w328:T1)
                n163 = property class="WFGraph (strict)"(reference=w320, "YScale.Minimum"=w317, "YScale.Maximum"=w316) -> ()  [unwired: 1 in, 2 out]
              }
              frame "Z-Axis" {
                # "Needed to update\nZ-axis markers"
                n164 = Unbundle By Name(w342) -> ("Z-Axis Range.Minimum"=w341:dbl, "Z-Axis Scaling Factor.Multiplier"=w338:dbl, "Z-Axis Range.Maximum"=w339:dbl)
                n165 = Generate User Event(user event=w333, event data cluster=svx_Waterfall_Property_Page_User_Events."Update Graph" ("event data")) -> ()  [unwired: 2 in, 2 out]
                n166 = Multiply(x=w341, y=w338) -> (x*y=w340:dbl)
                n167 = Multiply(x=w338, y=w339) -> (x*y=w337:dbl)
                n168 = Add(x=w336, y=w340) -> (x+y=w332:dbl)
                n169 = Add(x=w336, y=w337) -> (x+y=w329:dbl)
                n170 = Max & Min(x=w332, y=w329) -> (max(x,y)=w330:dbl, min(x,y)=w331:dbl)
                n171 = Bundle By Name(cluster=w342, "Z-Axis Scaling Factor.Offset"=w336, "Z-Axis Range Scaled.Minimum"=w331, "Z-Axis Range Scaled.Maximum"=w330) -> (w343:T1)
                n172 = property class="WFGraph (strict)"(reference=w335, "YScale.Minimum"=w331, "YScale.Maximum"=w330) -> ()  [unwired: 1 in, 2 out]
              }
            }
            n173 = Bundle By Name(cluster=w295, "Scales Changed"=TRUE) -> (w294:T8)
            n174 = local write "Range Minimum"(w298) -> ()
            n175 = local write "Range Maximum"(w297) -> ()
          }
          event "Scaling Factors - Multiplier": Value Change {
            n176 = event-data() -> ("NewVal"=w353:dbl)  [unwired: 1 in]
            n177 = local read "Scale Axis"() -> (w350:enum16{"X-Axis", "Y-Axis", "Z-Axis"})
            n178 = case shown="\"X-Axis\"" w350 {
              tunnel: w355 -> [w368 w382 w398]
              tunnel: [w369 w383 w399] -> w354
              tunnel: w353 -> [w360 w375 w385]
              tunnel: w352 -> [w362 w377 _]
              tunnel: w351 -> [_ _ w393]
              tunnel: [w357 w370 w386] -> w349
              tunnel: [w356 w371 w387] -> w348
              tunnel: w344 -> [_ _ w390]
              frame "X-Axis" {
                n179 = Unbundle By Name(w368) -> ("X-Axis Range.Minimum"=w367:dbl, "X-Axis Scaling Factor.Offset"=w363:dbl, "X-Axis Range.Maximum"=w365:dbl)
                n180 = Multiply(x=w360, y=w367) -> (x*y=w366:dbl)
                n181 = Multiply(x=w360, y=w365) -> (x*y=w364:dbl)
                n182 = Add(x=w366, y=w363) -> (x+y=w358:dbl)
                n183 = Add(x=w363, y=w364) -> (x+y=w359:dbl)
                n184 = Max & Min(x=w358, y=w359) -> (max(x,y)=w356:dbl, min(x,y)=w357:dbl)
                n185 = Bundle By Name(cluster=w368, "X-Axis Scaling Factor.Multiplier"=w360, "X-Axis Range Scaled.Maximum"=w356, "X-Axis Range Scaled.Minimum"=w357) -> (w369:T1)
                n186 = Less Than 0?(x=w360) -> (x < 0?=w361:bool)
                n187 = property class="WFGraph (strict)"(reference=w362, "XScale.Flipped"=w361, "XScale.Maximum"=w356, "XScale.Minimum"=w357) -> ()  [unwired: 1 in, 2 out]
              }
              frame "Y-Axis" {
                n188 = Unbundle By Name(w382) -> ("Y-Axis Range.Minimum"=w381:dbl, "Y-Axis Scaling Factor.Offset"=w376:dbl, "Y-Axis Range.Maximum"=w379:dbl)
                n189 = Multiply(x=w375, y=w381) -> (x*y=w380:dbl)
                n190 = Multiply(x=w375, y=w379) -> (x*y=w378:dbl)
                n191 = Add(x=w380, y=w376) -> (x+y=w373:dbl)
                n192 = Add(x=w376, y=w378) -> (x+y=w372:dbl)
                n193 = Max & Min(x=w373, y=w372) -> (max(x,y)=w371:dbl, min(x,y)=w370:dbl)
                n194 = Bundle By Name(cluster=w382, "Y-Axis Scaling Factor.Multiplier"=w375, "Y-Axis Range Scaled.Maximum"=w371, "Y-Axis Range Scaled.Minimum"=w370) -> (w383:T1)
                n195 = Less Than 0?(x=w375) -> (x < 0?=w374:bool)
                n196 = property class="WFGraph (strict)"(reference=w377, "YScale.Flipped"=w374, "YScale.Maximum"=w371, "YScale.Minimum"=w370) -> ()  [unwired: 1 in, 2 out]
              }
              frame "Z-Axis" {
                # "Needed to update\nZ-axis markers"
                n197 = Unbundle By Name(w398) -> ("Z-Axis Range.Minimum"=w397:dbl, "Z-Axis Scaling Factor.Offset"=w392:dbl, "Z-Axis Range.Maximum"=w395:dbl)
                n198 = Generate User Event(user event=w390, event data cluster=svx_Waterfall_Property_Page_User_Events."Update Graph" ("event data")) -> ()  [unwired: 2 in, 2 out]
                n199 = Multiply(x=w385, y=w397) -> (x*y=w396:dbl)
                n200 = Multiply(x=w385, y=w395) -> (x*y=w394:dbl)
                n201 = Add(x=w396, y=w392) -> (x+y=w389:dbl)
                n202 = Add(x=w392, y=w394) -> (x+y=w388:dbl)
                n203 = Less Than 0?(x=w385) -> (x < 0?=w384:bool)
                n204 = Max & Min(x=w389, y=w388) -> (max(x,y)=w387:dbl, min(x,y)=w386:dbl)
                n205 = Bundle By Name(cluster=w398, "Z-Axis Scaling Factor.Multiplier"=w385, "Z-Axis Range Scaled.Minimum"=w386, "Z-Axis Range Scaled.Maximum"=w387) -> (w399:T1)
                n206 = property class="WFGraph (strict)"(reference=w393, "YScale.Minimum"=w386, "YScale.Maximum"=w387, "YScale.Flipped"=w384) -> ()  [unwired: 1 in, 2 out]
              }
            }
            n207 = Bundle By Name(cluster=w346, "Scales Changed"=TRUE) -> (w345:T8)
            n208 = local write "Range Minimum"(w349) -> ()
            n209 = local write "Range Maximum"(w348) -> ()
          }
          event "Range Minimum": Value Change {
            n210 = event-data() -> ("NewVal"=w411:dbl)  [unwired: 1 in]
            n211 = local read "Scale Axis"() -> (w408:enum16{"X-Axis", "Y-Axis", "Z-Axis"})
            n212 = Generate User Event(user event=w406, event data cluster=svx_Waterfall_Property_Page_User_Events."Update Graph" ("event data")) -> ()  [unwired: 2 in, 2 out]
            n213 = case shown="\"Z-Axis\"" w408 {
              tunnel: w413 -> [w424 w436 w446]
              tunnel: [w425 w437 w447] -> w412
              tunnel: w411 -> [w419 w426 w443]
              tunnel: w410 -> [w423 w435 _]
              tunnel: w409 -> [_ _ _]
              tunnel: w407 -> [_ _ _]
              tunnel: [w417 w430 w445] -> w401
              tunnel: [w416 w429 w444] -> w400
              frame "X-Axis" {
                n214 = Unbundle By Name(w424) -> ("X-Axis Scaling Factor.Multiplier"=w422:dbl, "X-Axis Scaling Factor.Offset"=w421:dbl, "X-Axis Range Scaled.Maximum"=w420:dbl)
                n215 = call <vilib>:"svx_XYZ Scale.vi"("Minimum"=w419, "Maximum"=w420, "Offset"=w421, "Multiplier"=w422) -> ("Scaled.Minimum"=w416:dbl, "Scaled.Maximum"=w417:dbl, "Range.Minimum"=w414:dbl, "Range.Maximum"=w415:dbl, "flipped?"=w418:bool)  [unwired: 3 in]
                n216 = property class="WFGraph (strict)"(reference=w423, "XScale.Flipped"=w418) -> ()  [unwired: 1 in, 2 out]
                n217 = Bundle By Name(cluster=w424, "X-Axis Range.Maximum"=w415, "X-Axis Range.Minimum"=w414, "X-Axis Range Scaled.Maximum"=w417, "X-Axis Range Scaled.Minimum"=w416) -> (w425:T1)
              }
              frame "Y-Axis" {
                n218 = Unbundle By Name(w436) -> ("Y-Axis Scaling Factor.Multiplier"=w433:dbl, "Y-Axis Scaling Factor.Offset"=w432:dbl, "Y-Axis Range Scaled.Maximum"=w431:dbl)
                n219 = call <vilib>:"svx_XYZ Scale.vi"("Minimum"=w426, "Maximum"=w431, "Offset"=w432, "Multiplier"=w433) -> ("Scaled.Minimum"=w429:dbl, "Scaled.Maximum"=w430:dbl, "Range.Minimum"=w427:dbl, "Range.Maximum"=w428:dbl, "flipped?"=w434:bool)  [unwired: 3 in]
                n220 = Bundle By Name(cluster=w436, "Y-Axis Range.Maximum"=w428, "Y-Axis Range.Minimum"=w427, "Y-Axis Range Scaled.Maximum"=w430, "Y-Axis Range Scaled.Minimum"=w429) -> (w437:T1)
                n221 = property class="WFGraph (strict)"(reference=w435, "YScale.Flipped"=w434) -> ()  [unwired: 1 in, 2 out]
              }
              frame "Z-Axis" {
                n222 = Unbundle By Name(w446) -> ("Z-Axis Scaling Factor.Multiplier"=w440:dbl, "Z-Axis Scaling Factor.Offset"=w441:dbl, "Z-Axis Range Scaled.Maximum"=w442:dbl)
                n223 = call <vilib>:"svx_XYZ Scale.vi"("Minimum"=w443, "Maximum"=w442, "Offset"=w441, "Multiplier"=w440) -> ("Scaled.Minimum"=w444:dbl, "Scaled.Maximum"=w445:dbl, "Range.Minimum"=w438:dbl, "Range.Maximum"=w439:dbl)  [unwired: 3 in, 1 out]
                n224 = Bundle By Name(cluster=w446, "Z-Axis Range.Maximum"=w439, "Z-Axis Range.Minimum"=w438, "Z-Axis Range Scaled.Maximum"=w445, "Z-Axis Range Scaled.Minimum"=w444) -> (w447:T1)
              }
            }
            n225 = Bundle By Name(cluster=w403, "Scales Changed"=TRUE) -> (w402:T8)
            n226 = local write "Range Maximum"(w401) -> ()
            n227 = local write "Range Minimum"(w400) -> ()
          }
          event "Range Maximum": Value Change {
            n228 = event-data() -> ("NewVal"=w459:dbl)  [unwired: 1 in]
            n229 = local read "Scale Axis"() -> (w456:enum16{"X-Axis", "Y-Axis", "Z-Axis"})
            n230 = Generate User Event(user event=w454, event data cluster=svx_Waterfall_Property_Page_User_Events."Update Graph" ("event data")) -> ()  [unwired: 2 in, 2 out]
            n231 = case shown="\"X-Axis\"" w456 {
              tunnel: w461 -> [w472 w484 w494]
              tunnel: [w473 w485 w495] -> w460
              tunnel: w459 -> [w464 w474 w489]
              tunnel: w458 -> [w471 w483 _]
              tunnel: w457 -> [_ _ _]
              tunnel: w455 -> [_ _ _]
              tunnel: [w468 w480 w493] -> w449
              tunnel: [w469 w481 w492] -> w448
              frame "X-Axis" {
                n232 = Unbundle By Name(w472) -> ("X-Axis Scaling Factor.Multiplier"=w467:dbl, "X-Axis Scaling Factor.Offset"=w466:dbl, "X-Axis Range Scaled.Minimum"=w465:dbl)
                n233 = call <vilib>:"svx_XYZ Scale.vi"("Minimum"=w465, "Maximum"=w464, "Offset"=w466, "Multiplier"=w467) -> ("Scaled.Minimum"=w469:dbl, "Scaled.Maximum"=w468:dbl, "Range.Minimum"=w462:dbl, "Range.Maximum"=w463:dbl, "flipped?"=w470:bool)  [unwired: 3 in]
                n234 = property class="WFGraph (strict)"(reference=w471, "XScale.Flipped"=w470) -> ()  [unwired: 1 in, 2 out]
                n235 = Bundle By Name(cluster=w472, "X-Axis Range.Maximum"=w463, "X-Axis Range.Minimum"=w462, "X-Axis Range Scaled.Maximum"=w468, "X-Axis Range Scaled.Minimum"=w469) -> (w473:T1)
              }
              frame "Y-Axis" {
                n236 = Unbundle By Name(w484) -> ("Y-Axis Scaling Factor.Multiplier"=w477:dbl, "Y-Axis Scaling Factor.Offset"=w476:dbl, "Y-Axis Range Scaled.Minimum"=w475:dbl)
                n237 = call <vilib>:"svx_XYZ Scale.vi"("Minimum"=w475, "Maximum"=w474, "Offset"=w476, "Multiplier"=w477) -> ("Scaled.Minimum"=w481:dbl, "Scaled.Maximum"=w480:dbl, "Range.Minimum"=w478:dbl, "Range.Maximum"=w479:dbl, "flipped?"=w482:bool)  [unwired: 3 in]
                n238 = Bundle By Name(cluster=w484, "Y-Axis Range.Maximum"=w479, "Y-Axis Range.Minimum"=w478, "Y-Axis Range Scaled.Maximum"=w480, "Y-Axis Range Scaled.Minimum"=w481) -> (w485:T1)
                n239 = property class="WFGraph (strict)"(reference=w483, "YScale.Flipped"=w482) -> ()  [unwired: 1 in, 2 out]
              }
              frame "Z-Axis" {
                n240 = Unbundle By Name(w494) -> ("Z-Axis Scaling Factor.Multiplier"=w488:dbl, "Z-Axis Scaling Factor.Offset"=w486:dbl, "Z-Axis Range Scaled.Minimum"=w487:dbl)
                n241 = call <vilib>:"svx_XYZ Scale.vi"("Minimum"=w487, "Maximum"=w489, "Offset"=w486, "Multiplier"=w488) -> ("Scaled.Minimum"=w492:dbl, "Scaled.Maximum"=w493:dbl, "Range.Minimum"=w490:dbl, "Range.Maximum"=w491:dbl)  [unwired: 3 in, 1 out]
                n242 = Bundle By Name(cluster=w494, "Z-Axis Range.Maximum"=w491, "Z-Axis Range.Minimum"=w490, "Z-Axis Range Scaled.Maximum"=w493, "Z-Axis Range Scaled.Minimum"=w492) -> (w495:T1)
              }
            }
            n243 = Bundle By Name(cluster=w451, "Scales Changed"=TRUE) -> (w450:T8)
            n244 = local write "Range Maximum"(w449) -> ()
            n245 = local write "Range Minimum"(w448) -> ()
          }
          event "Autoscale": Value Change {
            n246 = event-data() -> ("NewVal"=w500:bool)  [unwired: 1 in]
            n247 = Generate User Event(user event=w505, event data cluster=svx_Waterfall_Property_Page_User_Events."Update Graph" ("event data")) -> ()  [unwired: 2 in, 2 out]
            n248 = local read "Scale Axis"() -> (w496:enum16{"X-Axis", "Y-Axis", "Z-Axis"})
            n249 = Select(t=u8 2, s=w500, f=u8 0 ("Disabled")) -> (s? t:f=w499:u8)
            n250 = case shown="\"X-Axis\"" w496 {
              tunnel: w507 -> [w510 w513 w516]
              tunnel: [w509 w512 w515] -> w506
              tunnel: w499 -> [w508 w511 w514]
              frame "X-Axis" {
                n251 = Bundle By Name(cluster=w510, "AutoScale X"=w508) -> (w509:T1)
              }
              frame "Y-Axis" {
                n252 = Bundle By Name(cluster=w513, "AutoScale Y"=w511) -> (w512:T1)
              }
              frame "Z-Axis" {
                n253 = Bundle By Name(cluster=w516, "AutoScale Z"=w514) -> (w515:T1)
              }
            }
            n254 = Bundle By Name(cluster=w502, "Scales Changed"=TRUE) -> (w501:T8)
            n255 = property on="Range Minimum" class="DigNum (strict)"("Disabled"=w499) -> ()  [unwired: 2 in, 2 out]
            n256 = property on="Range Maximum" class="DigNum (strict)"("Disabled"=w499) -> ()  [unwired: 2 in, 2 out]
          }
          event "FP Axis": Value Change {
            n257 = event-data() -> ("NewVal"=w519:enum16{"X-Axis", "Y-Axis", "Z-Axis"})  [unwired: 1 in]
            n258 = case shown="\"Y-Axis\"" w519 {
              tunnel: w518 -> [w526 w528 w530]
              tunnel: [w525 w527 w529] -> w517
              frame "X-Axis", Default {
                n259 = Unbundle By Name(w526) -> ("X-Scale Format Str"=w525:string)
              }
              frame "Y-Axis" {
                n260 = Unbundle By Name(w528) -> ("Y-Scale Format Str"=w527:string)
              }
              frame "Z-Axis" {
                n261 = Unbundle By Name(w530) -> ("Z-Scale Format Str"=w529:string)
              }
            }
            n262 = call <vilib>:"svx_Parse Format String.vi"("Format string"=w517) -> ("trailing zeros"=w522:bool, "Precision Type"=w523:u16, "Digits"=w524:u8, "Type"=w520:i32)  [unwired: 6 in, 1 out]
            n263 = local write "Type"(w520) -> ()
            n264 = local write "Precision Type"(w523) -> ()
            n265 = local write "trailing zeros"(w522) -> ()
            n266 = local write "Digits"(w524) -> ()
          }
          event "Type", "Precision Type", "Digits", "trailing zeros": Value Change {
            n267 = event-data() -> ()  [unwired: 1 in, 6 out]
            n268 = call <vilib>:"svx_Build Format String.vi"("trailing zeros"="trailing zeros", "Precision Type"="Precision Type", "Digits"="Digits", "Type"="Type") -> ("String"=w535:string)
            n269 = case shown="\"Z-Axis\"" "FP Axis" {
              tunnel: w539 -> [w547 w551 w555]
              tunnel: [w546 w550 w554] -> w540
              tunnel: w535 -> [w545 w548 w553]
              tunnel: w537 -> [w544 w549 _]
              tunnel: w536 -> [_ _ w552]
              frame "X-Axis" {
                n270 = Bundle By Name(cluster=w547, "X-Scale Format Str"=w545) -> (w546:T1)
                n271 = property class="WFGraph (strict)"(reference=w544, "XScale.FormatString"=w545) -> ()  [unwired: 1 in, 2 out]
              }
              frame "Y-Axis" {
                n272 = Bundle By Name(cluster=w551, "Y-Scale Format Str"=w548) -> (w550:T1)
                n273 = property class="WFGraph (strict)"(reference=w549, "YScale.FormatString"=w548) -> ()  [unwired: 1 in, 2 out]
              }
              frame "Z-Axis" {
                n274 = Bundle By Name(cluster=w555, "Z-Scale Format Str"=w553) -> (w554:T1)
                n275 = property class="WFGraph (strict)"(reference=w552, "YScale.FormatString"=w553) -> ()  [unwired: 1 in, 2 out]
              }
            }
            n276 = Bundle By Name(cluster=w542, "Scales Changed"=TRUE) -> (w541:T8)
          }
          event "OK": Value Change {
            w556 = FALSE
            n277 = event-data() -> ()  [unwired: 1 in, 1 out]
            n278 = Generate User Event(user event=w557, event data cluster=svx_Waterfall_Property_Page_User_Events."Exit" ("Property Page User Events")) -> ()  [unwired: 2 in, 2 out]
            n279 = local write "Cancel?"(w556) -> ()
          }
          event "Cancel": Value Change; Panel Close {
            n280 = event-data() -> ()  [unwired: 1 in, 1 out]
            n281 = stacked-sequence {
              tunnel: w569 -> [w573 w591 w609 _]
              tunnel: w568 -> [w571 _ _ _]
              tunnel: w567 -> [_ w589 _ w639]
              tunnel: w566 -> [_ w588 w605 _]
              tunnel: w565 -> [_ w587 _ _]
              tunnel: w564 -> [w570 _ _ _]
              tunnel: w563 -> [_ _ w607 _]
              tunnel: w562 -> [_ _ w606 _]
              tunnel: w561 -> [_ w583 _ _]
              frame #0 {
                n282 = Unbundle By Name(w573) -> ("Container Changed"=w572:bool)
                n283 = case shown="False" w572 {
                  tunnel: w571 -> [_ w582]
                  tunnel: w570 -> [_ w574]
                  frame False {
                  }
                  frame True {
                    n284 = Unbundle(w574) -> ("Label.Text"=w581:string, "Label.Visible"=w580:bool, "Caption.Text"=w579:string, "Caption.Visible"=w578:bool, "Disabled"=w577:u8, "Desc"=w576:string, "TipStrip"=w575:string)
                    n285 = property class="Ctl"(reference=w582, "Label.Text"=w581, "Label.Visible"=w580, "Caption.Text"=w579, "Caption.Visible"=w578, "Disabled"=w577, "Desc"=w576, "TipStrip"=w575) -> ()  [unwired: 1 in, 2 out]
                  }
                }
              }
              frame #1 {
                n286 = Unbundle By Name(w591) -> ("Waveform Changed"=w590:bool)
                n287 = Unbundle By Name(w588) -> ("Plot Transparency"=w584:bool, "Background Color"=w586:u32, "Plot Color"=w585:u32)
                n288 = case shown="True" w590 {
                  tunnel: w589 -> [_ w600]
                  tunnel: w587 -> [_ w592]
                  tunnel: w586 -> [_ w593]
                  tunnel: w585 -> [_ w598]
                  tunnel: w584 -> [_ w597]
                  tunnel: w583 -> [_ w594]
                  frame False {
                  }
                  frame True {
                    n289 = Select(t=u32 16777216, s=w597, f=w593) -> (s? t:f=w595:u32)
                    n290 = for {
                      N: w594 -> [_]
                      tunnel: w592 -> [w603]
                      tunnel: w595 -> [w601]
                      tunnel: w598 -> [w602]
                      i -> [w604]
                      n291 = property class="XYGraph (strict)"(reference=w603, "Active Plot"=w604, "Plot.Fill/Pt. Color"=w601, "Plot.Plot Color"=w602) -> ()  [unwired: 1 in, 2 out]
                    }
                    n292 = property class="XYGraph (strict)"(reference=w592, "BG Color"=w593) -> ()  [unwired: 1 in, 2 out]
                    n293 = Generate User Event(user event=w600, event data cluster=svx_Waterfall_Property_Page_User_Events."Redraw Frame" ("Property Page User Events")) -> ()  [unwired: 2 in, 2 out]
                  }
                }
              }
              frame #2 {
                n294 = Unbundle By Name(w609) -> ("Scales Changed"=w608:bool)
                n295 = case shown="True" w608 {
                  tunnel: w607 -> [_ w625]
                  tunnel: w606 -> [_ w629]
                  tunnel: w605 -> [_ w636]
                  frame False {
                  }
                  frame True {
                    n296 = Unbundle By Name(w636) -> ("X-Axis Scaling Factor.Multiplier"=w624:dbl, "Y-Axis Scaling Factor.Multiplier"=w622:dbl, "X-Axis Range Scaled.Minimum"=w635:dbl, "X-Axis Range Scaled.Maximum"=w634:dbl, "X-Axis Name"=w633:string, "Y-Axis Range Scaled.Minimum"=w632:dbl, "Y-Axis Range Scaled.Maximum"=w631:dbl, "Y-Axis Name"=w630:string, "X-Scale Visible"=w619:bool, "Y-Scale Visible"=w620:bool, "X-Scale Label Visible"=w616:bool, "Y-Scale Label Visible"=w617:bool, "X-Scale Format Str"=w614:string, "Y-Scale Format Str"=w613:string, "Z-Axis Range Scaled.Minimum"=w628:dbl, "Z-Axis Range Scaled.Maximum"=w627:dbl, "Z-Axis Name"=w626:string, "Z-Scale Visible"=w618:bool, "Z-Scale Label Visible"=w615:bool, "Z-Scale Format Str"=w612:string, "Z-Axis Scaling Factor.Multiplier"=w611:dbl)
                    n297 = Less Than 0?(x=w611) -> (x < 0?=w610:bool)
                    n298 = Less Than 0?(x=w624) -> (x < 0?=w623:bool)
                    n299 = Less Than 0?(x=w622) -> (x < 0?=w621:bool)
                    n300 = property class="WFGraph (strict)"(reference=w625, "XScale.Flipped"=w623, "YScale.Flipped"=w621, "XScale.Minimum"=w635, "XScale.Maximum"=w634, "XScale.NameLbl.Text"=w633, "YScale.Minimum"=w632, "YScale.Maximum"=w631, "YScale.NameLbl.Text"=w630, "XScale.Visible"=w619, "YScale.Visible"=w620, "XScale.NameLbl.Visible"=w616, "YScale.NameLbl.Visible"=w617, "XScale.FormatString"=w614, "YScale.FormatString"=w613) -> ()  [unwired: 1 in, 2 out]
                    n301 = property class="WFGraph (strict)"(reference=w629, "YScale.Minimum"=w628, "YScale.Maximum"=w627, "YScale.NameLbl.Text"=w626, "YScale.Visible"=w618, "YScale.NameLbl.Visible"=w615, "YScale.FormatString"=w612, "YScale.Flipped"=w610) -> ()  [unwired: 1 in, 2 out]
                  }
                }
              }
              frame #3 {
                n302 = Generate User Event(user event=w639, event data cluster=svx_Waterfall_Property_Page_User_Events."Exit" ("Property Page User Events")) -> ()  [unwired: 2 in, 2 out]
                "Cancel?" <- "Cancel"
              }
            }
          }
          event "Help": Value Change {
            n303 = event-data() -> ()  [unwired: 1 in, 1 out]
            n304 = Control Online Help(2:path "<helpdir>/sndvibtk.chm" ("Path to the help file"), 3:"Waterfall_Graph_Prop_DB.html" ("String to search for"), 4:enum16{"Contents", "Key", "Close"}."Key" ("Operation")) -> ()  [unwired: 1 in, 1 out]
          }
          event User Event {
            n305 = event-data() -> ("Property Page User Events"=w653:T7)  [unwired: 1 in]
            n306 = case shown="\"Update Graph\"" w653 {
              tunnel: [_ _ TRUE] -> w652
              tunnel: w651 -> [w684 w714 _]
              tunnel: w650 -> [w683 w704 _]
              tunnel: w649 -> [_ w708 _]
              tunnel: w648 -> [w680 w706 w725]
              tunnel: w647 -> [_ _ w726]
              tunnel: w646 -> [_ w699 _]
              tunnel: [w680 w696 w725] -> w645
              frame "Redraw Frame", Default {
                w655 = cluster{"x":i16, "y":i16} {"x"=0, "y"=0} ("cluster")
                w665 = u32 0 ("Offset")
                w686 = T11 {"Width"=1, "Style"=enum."Solid"} ("pen")
                n307 = property class="WFGraph (strict)"(reference=w683) -> ("Width"=w663:u32, "Height"=w658:u32)  [unwired: 1 in, 2 out]
                n308 = property class="XYGraph (strict)"(reference=w684) -> (reference out=w682:refnum<vi>, "Width"=w662:u32, "Height"=w659:u32)  [unwired: 1 in, 1 out]
                n309 = Unbundle By Name(w680) -> ("Frame Color"=w681:u32)
                n310 = Subtract(x=w662, y=w663) -> (x-y=w669:u32)
                n311 = Subtract(x=w659, y=w658) -> (x-y=w660:u32)
                n312 = Increment(x=w662) -> (x+1=w661:u32)
                n313 = Decrement(x=w658) -> (x-1=w670:u32)
                n314 = Increment(x=w669) -> (x+1=w668:u32)
                n315 = Decrement(x=w665) -> (x-1=w666:u32)
                n316 = Decrement(x=w660) -> (x-1=w667:u32)
                n317 = Increment(x=w665) -> (x+1=w664:u32)
                n318 = Decrement(x=w659) -> (x-1=w673:u32)
                n319 = Increment(x=w663) -> (x+1=w672:u32)
                n320 = Decrement(x=w659) -> (x-1=w671:u32)
                n321 = Bundle(cluster=w655, "x"=w661, "y"=w670) -> (w674:cluster{"x":i16, "y":i16})
                n322 = Bundle(cluster=w655, "x"=w668, "y"=w670) -> (w675:cluster{"x":i16, "y":i16})
                n323 = Bundle(cluster=w655, "x"=w668, "y"=w666) -> (w679:cluster{"x":i16, "y":i16})
                n324 = Bundle(cluster=w655, "x"=w664, "y"=w667) -> (w678:cluster{"x":i16, "y":i16})
                n325 = Bundle(cluster=w655, "x"=w664, "y"=w673) -> (w676:cluster{"x":i16, "y":i16})
                n326 = Bundle(cluster=w655, "x"=w672, "y"=w671) -> (w677:cluster{"x":i16, "y":i16})
                n327 = Build Array(w674, w675, w679, w678, w676, w675) -> (w656:cluster{"x":i16, "y":i16}[])
                n328 = Build Array(w676, w677, w674) -> (w657:cluster{"x":i16, "y":i16}[])
                n329 = call <vilib>:"Draw Multiple Lines.vi"("line endpoints"=w656, "color(black)"=w681, "pen"=w686) -> ("new picture"=w685:picture)  [unwired: 6 in]
                n330 = call <vilib>:"Draw Multiple Lines.vi"("line endpoints"=w657, "color(black)"=w681, "pen"=w686) -> ("new picture"=w687:picture)  [unwired: 6 in]
                n331 = property on="Property Node" class="XYGraph (strict)"(reference=w682, "PlotImages.Back"=w685, "PlotImages.Front"=w687) -> ()  [unwired: 1 in, 2 out]
              }
              frame "Update Graph" {
                n332 = call <vilib>:"svx_Autoscale Ranges.vi"("Display State In"=w706, "Data Array In"=w708) -> ("Cropped Info out"=w690:cluster{"First Index":i32, "Length":i32}, "Display State Out"=w705:T1, "Dec/Cropped and Lines Out"=w715:T12)  [unwired: 5 in, 2 out]
                n333 = local read "Scale Axis"() -> (w707:enum16{"X-Axis", "Y-Axis", "Z-Axis"})
                n334 = call <vilib>:"svx_Fit Data to Scale.vi"("Cropped Info"=w690, "Display State In"=w705, "Data In"=w715) -> ("Waveform YScale Max"=w710:dbl, "Waveform XScale Max"=w711:dbl, "Display State Out"=w696:T1, "Data Out"=w709:T12, "Markers"=w691:dbl[])  [unwired: 2 in, 2 out]
                n335 = Unbundle By Name(w696) -> ("X-Axis Range Scaled.Minimum"=w703:dbl, "X-Axis Range Scaled.Maximum"=w702:dbl, "Y-Axis Range Scaled.Minimum"=w701:dbl, "Y-Axis Range Scaled.Maximum"=w700:dbl, "Z-Axis Range Scaled.Minimum"=w698:dbl, "Z-Axis Range Scaled.Maximum"=w697:dbl)
                n336 = case shown="\"X-Axis\"" w707 {
                  tunnel: [w718 w721 w724] -> w695
                  tunnel: [w717 w720 w723] -> w694
                  tunnel: w696 -> [w716 w719 w722]
                  frame "X-Axis" {
                    n337 = Unbundle By Name(w716) -> ("X-Axis Range Scaled.Minimum"=w718:dbl, "X-Axis Range Scaled.Maximum"=w717:dbl)
                  }
                  frame "Y-Axis" {
                    n338 = Unbundle By Name(w719) -> ("Y-Axis Range Scaled.Minimum"=w721:dbl, "Y-Axis Range Scaled.Maximum"=w720:dbl)
                  }
                  frame "Z-Axis" {
                    n339 = Unbundle By Name(w722) -> ("Z-Axis Range Scaled.Minimum"=w724:dbl, "Z-Axis Range Scaled.Maximum"=w723:dbl)
                  }
                }
                n340 = Unbundle By Name(w709) -> ("Dec/Cropped in.Plots"=w689:cluster{"x0":dbl, "dx":dbl, "Y":dbl[]}[])
                n341 = Unbundle By Name(w696) -> ("X-Axis Range.Minimum"=w713:dbl, "Y-Axis Range.Minimum"=w712:dbl)
                n342 = call <vilib>:"svx_Convert Waveform Graph Data to XY Graph Data.vi"("Waveform Graph"=w689) -> ("XY Graph"=w688:cluster{"X":dbl[], "Y":dbl[]}[])  [unwired: 10 in]
                n343 = property on="Property Node" class="WFGraph (strict)"(reference=w704, "XScale.Minimum"=w703, "XScale.Maximum"=w702, "YScale.Minimum"=w701, "YScale.Maximum"=w700) -> ()  [unwired: 1 in, 2 out]
                n344 = property on="Property Node" class="WFGraph (strict)"(reference=w699, "YScale.Minimum"=w698, "YScale.Maximum"=w697, "YScale.MarkerVals[]"=w691) -> ()  [unwired: 1 in, 2 out]
                n345 = property on="Property Node" class="XYGraph (strict)"(reference=w714, "XScale.Minimum"=w713, "YScale.Minimum"=w712, "XScale.Maximum"=w711, "YScale.Maximum"=w710, "Value"=w688) -> ()  [unwired: 1 in, 2 out]
                n346 = Max & Min(x=w695, y=w694) -> (max(x,y)=w693:dbl, min(x,y)=w692:dbl)
                n347 = local write "Range Maximum"(w693) -> ()
                n348 = local write "Range Minimum"(w692) -> ()
              }
              frame "Exit" {
                n349 = Destroy User Event(user event=w726) -> ()  [unwired: 1 in, 1 out]
              }
            }
          }
          event "Line color", "Line width", "Style", "DisplayLines": Value Change {
            n350 = event-data() -> ()  [unwired: 1 in, 1 out]
            n351 = Bundle By Name(cluster=w733, "Line Properties.Line Color"="Line color", "Line Properties.Line Width"="Line width", "Line Properties.Line Style"="Style", "Line Properties.DisplayLines"="DisplayLines") -> (w732:T1)
          }
        }
      }
    }
  }
  "State out" <- w8
